vi "Read.vi"(8 "error in (no error)":errorcluster, 11 "Double Array in":refnum<class "Double Array.lvclass">) -> (0 "error out":errorcluster, 2 "Double Array":dbl[](array[numeric]), 3 "Double Array out":refnum<class "Double Array.lvclass">)   [LabVIEW 2020, in "Data.lvlib" / "Double Array.lvclass"]
doc: "Read Double Array."
uses:
  Double Array.lvclass
  Double Array.lvclass/Double Array.ctl
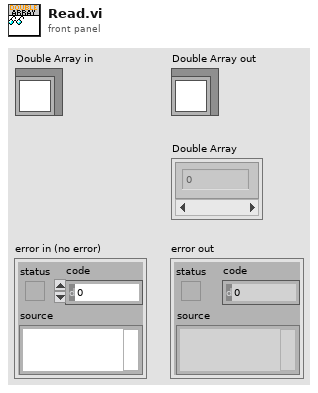
[diagram p1: front panel]
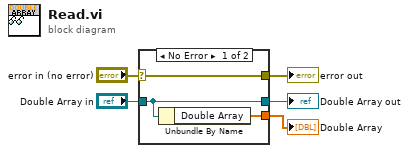
[diagram p0: block diagram]
diagram:
  n1 = case shown="No Error" "error in (no error)" {
    selector: "error in (no error)" -> [w8 w9]
    tunnel: [w8 w9] -> w4
    tunnel: [w7 w10] -> w2
    tunnel: "Double Array in" -> [w7 w10]
    tunnel: [w6 _] -> w1
    frame No Error {
      n2 = Unbundle By Name(w7) -> ("Double Array"=w6:dbl[])
    }
    frame Error {
    }
  }
  "error out" <- w4
  "Double Array out" <- w2
  "Double Array" <- w1
